vi "VIPT to rename.vi"(8 "error in (no error)":errorcluster, 11 "Package Source Folder":path) -> (0 "error out":errorcluster)   [LabVIEW 2019]
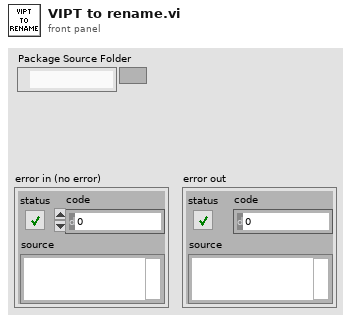
[diagram p1: front panel]
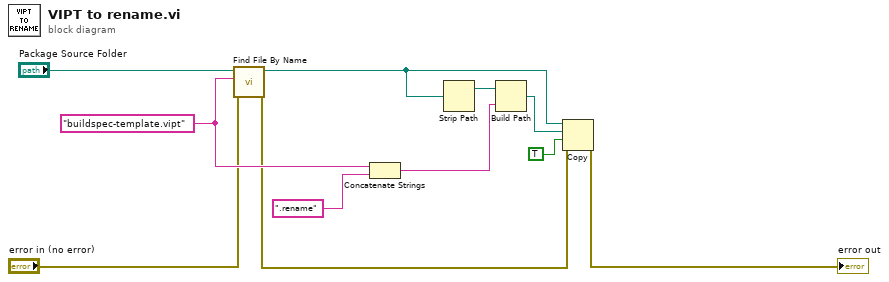
[diagram p0: block diagram]
diagram:
  w6 = "buildspec-template.vipt" ("name or relative path")
  n1 = call "Find File By Name.vi"("error in (no error)"="error in (no error)", "File Name"=w6, "Folder Path"="Package Source Folder") -> ("error out"=w2:errorcluster, "File Path"=w9:path)  [unwired: 7 in]
  n2 = Concatenate Strings(w6, ".rename" ("name or relative path")) -> (w7:string)
  n3 = Strip Path(path=w9) -> (stripped path=w8:path)  [unwired: 1 out]
  n4 = Build Path(base path=w8, name or relative path=w7) -> (appended path=w4:path)
  n5 = Copy(8:w2, 9:TRUE ("overwrite (F)"), 10:w4, 11:w9) -> (0:→"error out":errorcluster)  [unwired: 1 in, 2 out]
